vi "Merge Sort ACNET Device Arrays.vi"(0 "ACNET Device Array A":refnum<class "ACNET Device.lvclass">[](array[class]), 1 "Ignore Duplicates? (F)":bool=TRUE, 3 "ACNET Device Array B":refnum<class "ACNET Device.lvclass">[](array[class])) -> (6 "Sorted ACNET Device Array":refnum<class "ACNET Device.lvclass">[](array[class]))   [LabVIEW 2013]
uses:
  MTA Shift Toolbox/ACNET Monitor/ACNET Device.lvclass
panel:
  out "A Index":i32
  out "B Index":i32
  out "B Count":i32
  out "A Count":i32
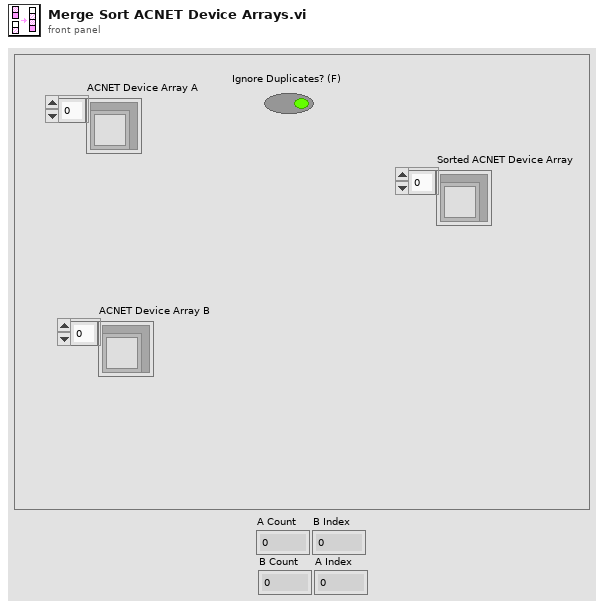
[diagram p1: front panel]
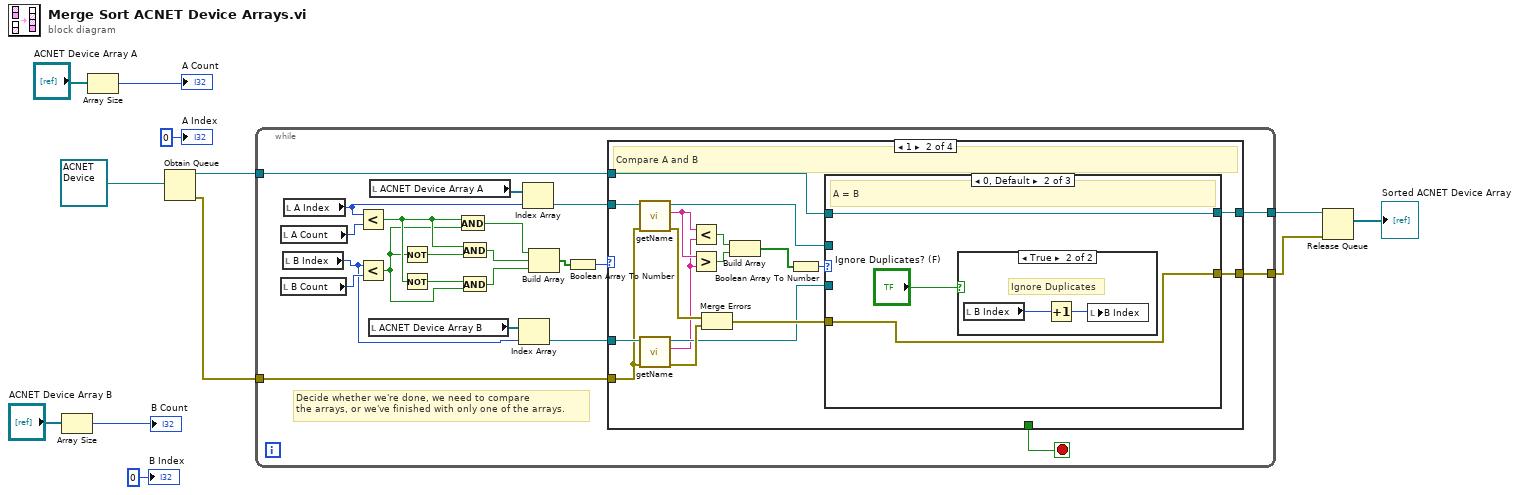
[diagram p0: block diagram]
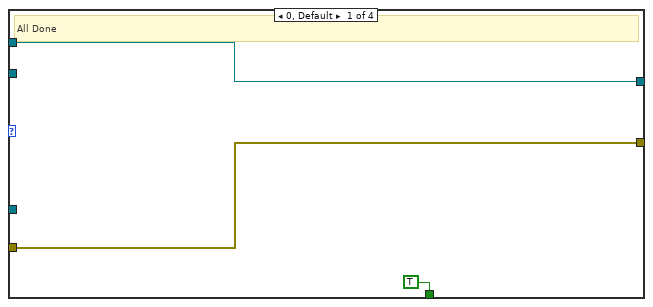
[diagram p2: hidden frame]
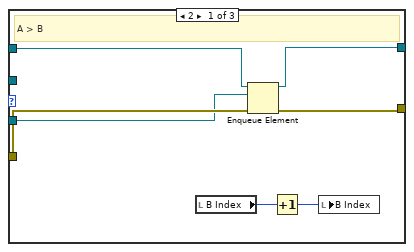
[diagram p3: hidden frame]
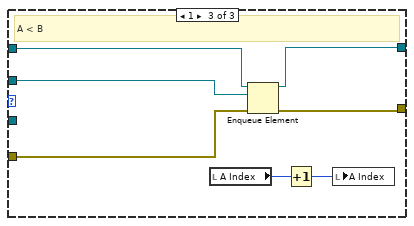
[diagram p5: hidden frame]
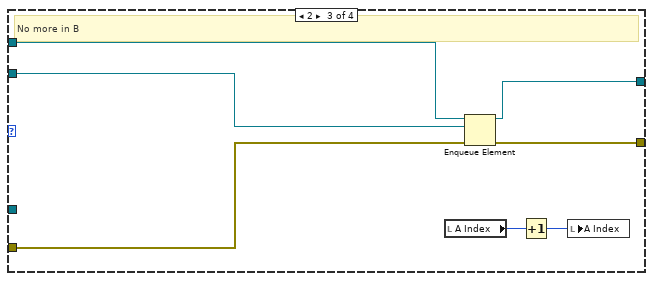
[diagram p6: hidden frame]
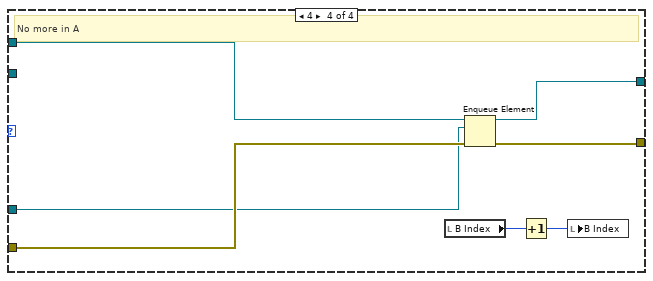
[diagram p7: hidden frame]
diagram:
  n1 = Array Size(array="ACNET Device Array B") -> (size(s)=→"B Count":i32)
  n2 = Array Size(array="ACNET Device Array A") -> (size(s)=→"A Count":i32)
  n3 = Obtain Queue(element data type=refnum<class "ACNET Device.lvclass"> refnum ("ACNET Device.lvclass")) -> (queue out=w11:refnum<queue>, error out=w10:errorcluster)  [unwired: 4 in, 1 out]
  n4 = while {
    tunnel: w11 -> [w23]
    tunnel: [w22] -> w3
    tunnel: [w21] -> w12
    tunnel: w10 -> [w20]
    stop <- w13 stop-if-true
    # "Decide whether we're done, we need to compare\nthe arrays, or we've finished with only one of the arrays."
    n5 = local read "A Count"() -> (w34:i32)
    n6 = local read "B Count"() -> (w33:i32)
    n7 = local read "B Index"() -> (w16:i32)
    n8 = local read "A Index"() -> (w18:i32)
    n9 = Less?(x=w18, y=w34) -> (x < y?=w30:bool)
    n10 = Less?(x=w16, y=w33) -> (x < y?=w29:bool)
    n11 = local read "ACNET Device Array B"() -> (w17:refnum<class "ACNET Device.lvclass">[])
    n12 = local read "ACNET Device Array A"() -> (w19:refnum<class "ACNET Device.lvclass">[])
    n13 = Not(x=w29) -> (.not. x?=w27:bool)
    n14 = Not(x=w30) -> (.not. x?=w26:bool)
    n15 = And(x=w30, y=w29) -> (x .and. y?=w32:bool)
    n16 = And(x=w30, y=w27) -> (x .and. y?=w31:bool)
    n17 = And(x=w26, y=w29) -> (x .and. y?=w28:bool)
    n18 = Index Array(array=w17, index=w16) -> (element=w15:refnum<class "ACNET Device.lvclass">)
    n19 = Index Array(array=w19, index=w18) -> (element=w14:refnum<class "ACNET Device.lvclass">)
    n20 = Build Array(w32, w31, w28) -> (w25:bool[])
    n21 = Boolean Array To Number(Boolean array=w25) -> (number=w24:u32)
    n22 = case shown="1" w24 {
      tunnel: w23 -> [w37 w54 w80 w87]
      tunnel: w14 -> [_ w51 w78 _]
      tunnel: w15 -> [_ w50 _ w85]
      tunnel: w20 -> [w36 w49 w79 w86]
      tunnel: [w36 w53 w76 w83] -> w22
      tunnel: [w37 w52 w77 w84] -> w21
      tunnel: [TRUE _ _ _] -> w13
      frame 0, Default {
        # "All Done"
      }
      frame 1 {
        # "Compare A and B"
        n23 = call-dynamic "getName.vi"("error in (no error)"=w49, "ACNET Device in"=w51) -> ("error out"=w47:errorcluster, "name"=w43:string, "ACNET Device out"=w44:refnum<class "ACNET Device.lvclass">)  [unwired: 7 in]
        n24 = call-dynamic "getName.vi"("error in (no error)"=w49, "ACNET Device in"=w50) -> ("error out"=w46:errorcluster, "name"=w42:string, "ACNET Device out"=w45:refnum<class "ACNET Device.lvclass">)  [unwired: 7 in]
        n25 = Less?(x=w43, y=w42) -> (x < y?=w41:bool)
        n26 = Greater?(x=w43, y=w42) -> (0:w40:bool)
        n27 = Merge Errors(w47, w46) -> (w48:errorcluster)
        n28 = Build Array(w41, w40) -> (w39:bool[])
        n29 = Boolean Array To Number(Boolean array=w39) -> (number=w38:u32)
        n30 = case shown="0, Default" w38 {
          tunnel: w54 -> [w61 w62 w73]
          tunnel: w44 -> [_ _ w72]
          tunnel: w45 -> [w55 _ _]
          tunnel: w48 -> [w60 w63 w71]
          tunnel: [w58 w63 w69] -> w53
          tunnel: [w59 w62 w70] -> w52
          frame 2 {
            # "A > B"
            n31 = local read "B Index"() -> (w56:i32)
            n32 = Enqueue Element(queue=w61, element=w55, error in (no error)=w60) -> (queue out=w59:refnum<queue>, error out=w58:errorcluster)  [unwired: 1 in, 1 out]
            n33 = Increment(x=w56) -> (x+1=w57:i32)
            n34 = local write "B Index"(w57) -> ()
          }
          frame 0, Default {
            # "A = B"
            n35 = case shown="True" "Ignore Duplicates? (F)" {
              frame False {
              }
              frame True {
                # "Ignore Duplicates"
                n36 = local read "B Index"() -> (w66:i32)
                n37 = Increment(x=w66) -> (x+1=w65:i32)
                n38 = local write "B Index"(w65) -> ()
              }
            }
          }
          frame 1 {
            # "A < B"
            n39 = local read "A Index"() -> (w67:i32)
            n40 = Enqueue Element(queue=w73, element=w72, error in (no error)=w71) -> (queue out=w70:refnum<queue>, error out=w69:errorcluster)  [unwired: 1 in, 1 out]
            n41 = Increment(x=w67) -> (x+1=w68:i32)
            n42 = local write "A Index"(w68) -> ()
          }
        }
      }
      frame 2 {
        # "No more in B"
        n43 = local read "A Index"() -> (w74:i32)
        n44 = Enqueue Element(queue=w80, element=w78, error in (no error)=w79) -> (queue out=w77:refnum<queue>, error out=w76:errorcluster)  [unwired: 1 in, 1 out]
        n45 = Increment(x=w74) -> (x+1=w75:i32)
        n46 = local write "A Index"(w75) -> ()
      }
      frame 4 {
        # "No more in A"
        n47 = local read "B Index"() -> (w81:i32)
        n48 = Enqueue Element(queue=w87, element=w85, error in (no error)=w86) -> (queue out=w84:refnum<queue>, error out=w83:errorcluster)  [unwired: 1 in, 1 out]
        n49 = Increment(x=w81) -> (x+1=w82:i32)
        n50 = local write "B Index"(w82) -> ()
      }
    }
  }
  n51 = Release Queue(queue=w12, error in (no error)=w3) -> (remaining elements=→"Sorted ACNET Device Array":refnum<class "ACNET Device.lvclass">[])  [unwired: 1 in, 2 out]
  "A Index" <- 0 ("A Index")
  "B Index" <- 0 ("B Index")
